vi "Sin.vi"() -> ()   [LabVIEW 2011]
uses:
  Control sin.ctl
panel:
  in  "stop":bool
  out "Waveform Chart":dbl(graph)
  in  "Exit":bool
  in  "Start":bool
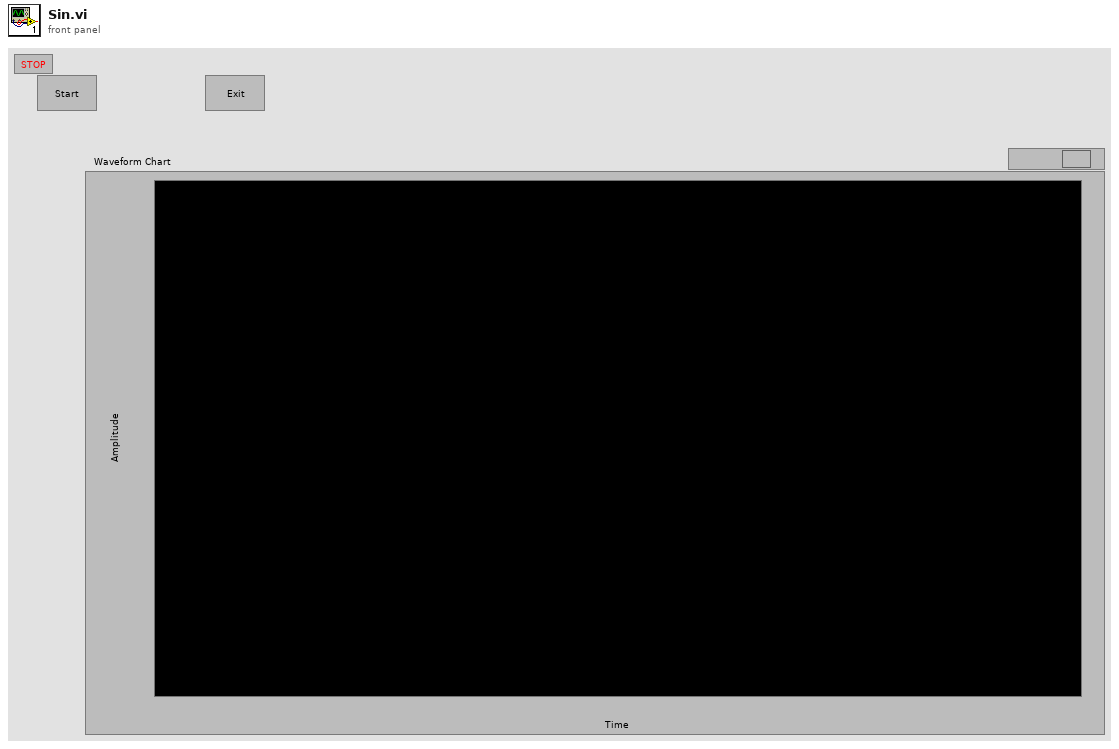
[diagram p1: front panel]
types:
  T1 = typedef "Control sin.ctl" = enum16{"Start", "Stop", "Exit", ""}
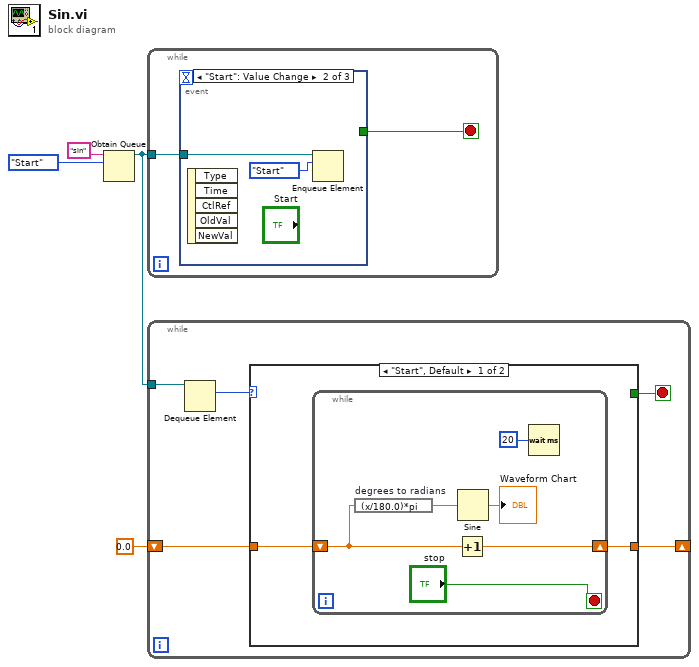
[diagram p0: block diagram]
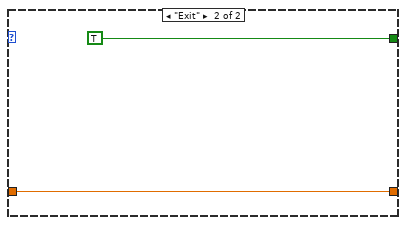
[diagram p2: hidden frame]
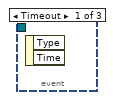
[diagram p3: hidden frame]
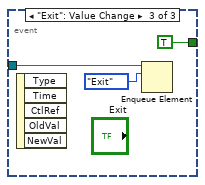
[diagram p4: hidden frame]
diagram:
  n1 = Obtain Queue(name (unnamed)="sin", element data type=Control_sin."Start" ("Enum")) -> (queue out=w2:refnum<queue>)  [unwired: 3 in, 2 out]
  n2 = while {
    tunnel: w2 -> [w6]
    stop <- w5 stop-if-true
    n3 = event shown="[1] \"Start\": Value Change" {
      selector: _ -> [_ _ _]
      dyn-events: _ -> [_ _ _]
      timeout: _ -> [_ _ _]
      tunnel: w6 -> [_ w8 w10]
      tunnel: [_ _ TRUE] -> w5
      event Timeout {
        n4 = event-data() -> ()  [unwired: 1 in, 2 out]
      }
      event "Start": Value Change {
        n5 = event-data() -> ()  [unwired: 1 in, 5 out]
        n6 = Enqueue Element(queue=w8, element=Control_sin."Start" ("Enum")) -> ()  [unwired: 2 in, 3 out]
      }
      event "Exit": Value Change {
        n7 = event-data() -> ()  [unwired: 1 in, 5 out]
        n8 = Enqueue Element(queue=w10, element=Control_sin."Exit" ("Enum")) -> ()  [unwired: 2 in, 3 out]
      }
    }
  }
  n9 = while {
    tunnel: w2 -> [w16]
    shift-right: [w12] -> _
    shift-left: 0.0 -> [w14]
    stop <- w13 stop-if-true
    n10 = Dequeue Element(queue=w16) -> (element=w15:T1)  [unwired: 2 in, 3 out]
    n11 = case shown="\"Start\", Default" w15 {
      tunnel: w14 -> [w18 w26]
      tunnel: [w17 w26] -> w12
      tunnel: [_ TRUE] -> w13
      frame "Start", Default {
        n12 = while {
          shift-right: [w19] -> w17
          shift-left: w18 -> [w20]
          stop <- "stop" stop-if-true
          n13 = expression code="(x/180.0)*pi" "degrees to radians"(w20) -> (w22:dbl)
          n14 = Increment(x=w20) -> (x+1=w19:dbl)
          n15 = Sine(x=w22) -> (sin(x)=→"Waveform Chart":dbl)
          n16 = Wait (ms)(milliseconds to wait=u32 20) -> ()  [unwired: 1 out]
        }
      }
      frame "Exit" {
      }
    }
  }
